vi "LowMaster.vi"() -> ()   [LabVIEW 2019]
uses:
  Ctl/tree.ctl
  Ctl/commands.ctl
  Ctl/Data Acquisition System.ctl
  Ctl/magnet.ctl
  Ctl/option.ctl
  <vilib>/Utility/file.llb/Write To Spreadsheet File (string).vi
panel:
  in  "Tab Control":T1(tab)
  in  "list":i32[](listbox)=[0]
  in  "Run":bool caption="Run/Stop"
  in  "open":bool
  in  "save":bool
  in  "copy 2":bool
  in  "paste":bool
  in  "delete":bool
  in  "clear":bool
  in  "Replace":bool
  in  "Update Sequence":bool
  in  "Tree":T2
  in  "line from":i32 caption="from line #" min=0
  out "log":i32[](listbox)
  in  "log save":bool
  in  "stop":bool
  out "Numeric":i32
  in  "Magnet":T3=enum."Cell8"
  in  "Data Acq":T4=enum."NML Data Acquisition-New.vi"
  in  "Quit LowMaster":bool
  out "current":i32
  in  "command":T5=enum."Comments"
  out "copy":string[][](array[string])
  # "Low Master 2016NT"
  # "Sequence Control Program   (contact: Ju-Hyun Park   JHPARK@magnet.fsu.edu)"
  # "Powered by MagLab"
  # "Magnet"
  # "QUIT LowMaster"
  # "Data Acquisition:"
  # "It doesn't hurt."
  # "Run/Stop"
  # "Sequence File"
  # "Sequence Edit Tool"
  # "* By default the log file is saved at the end of each run in the data folder."
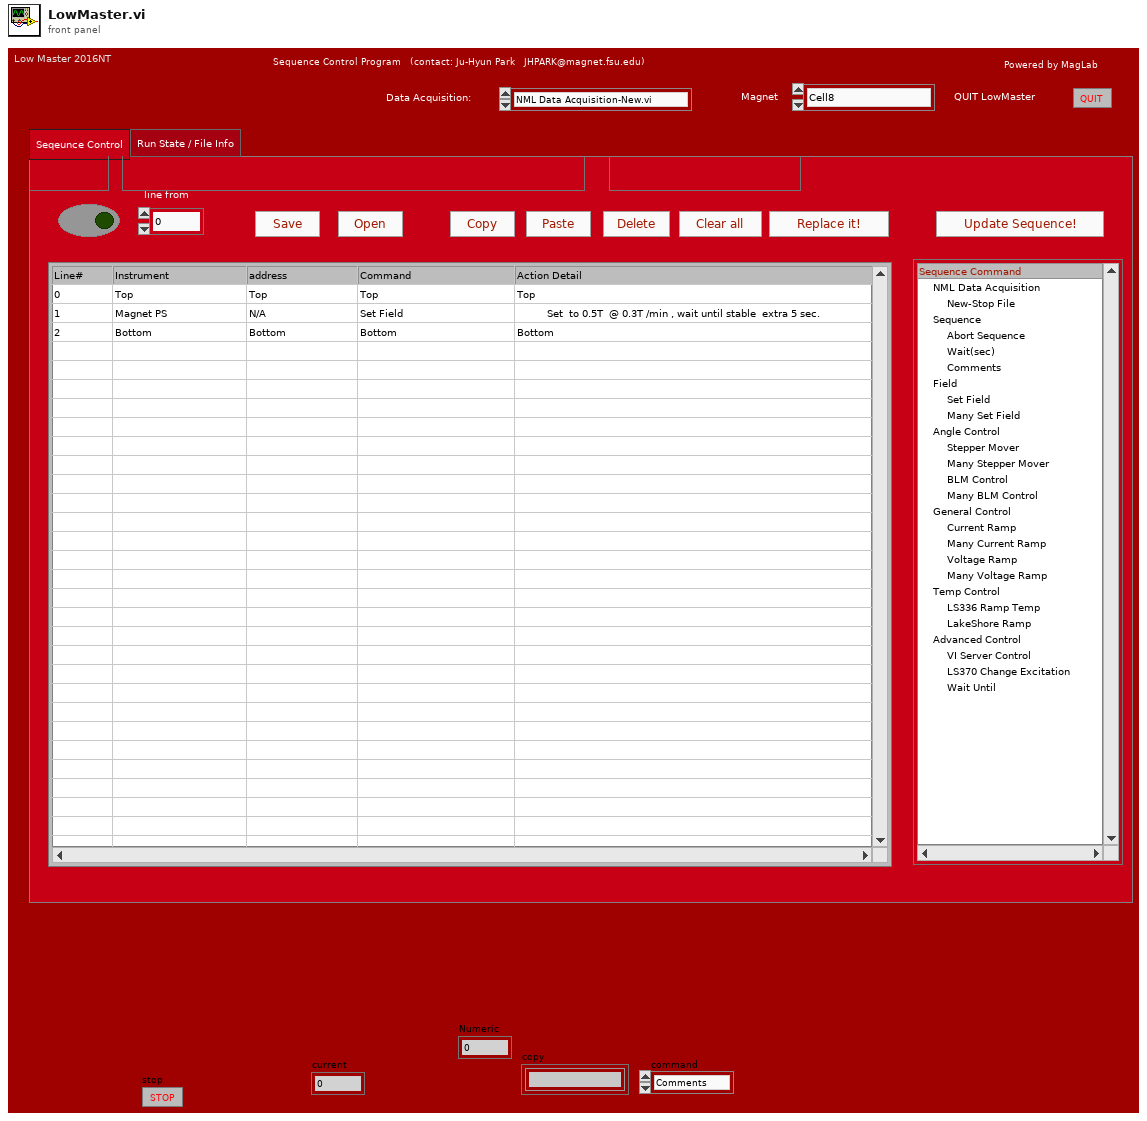
[diagram p1: front panel]
types:
  T1 = enum32{"Seqeunce Control", "Run State / File Info"}
  T2 = typedef "tree.ctl" = string[]
  T3 = typedef "magnet.ctl" = enum16{"SCM1", "SCM2", "SCM3", "SCMX", "Cell8", "Cell9", "Cell12", "Hybrid", "Great Magnet"}
  T4 = typedef "Data Acquisition System.ctl" = enum16{"NML Data Acquisition-old.vi", "NML Data Acquisition-New.vi"}
  T5 = typedef "commands.ctl" = enum16{"Voltage Ramp", "Many Voltage Ramp", "Current Ramp", "Many Current Ramp", "Comments", "Set Field", "Many Set Field", "Abort Sequence", "New-Stop File", "Wait(sec)", "BLM Control", "Many BLM Control", "Stepper Mover", "Many Stepper Mover", "LS336 Ramp Temp", "LakeShore Ramp", "VI Server Control", "LS370 Change Excitation", "Wait Until", "Nothing"}
  T6 = enum8{"Enabled", "Disabled", "Disabled and Grayed Out"}
  T7 = typedef "option.ctl" = enum16{"Tree", "List"}
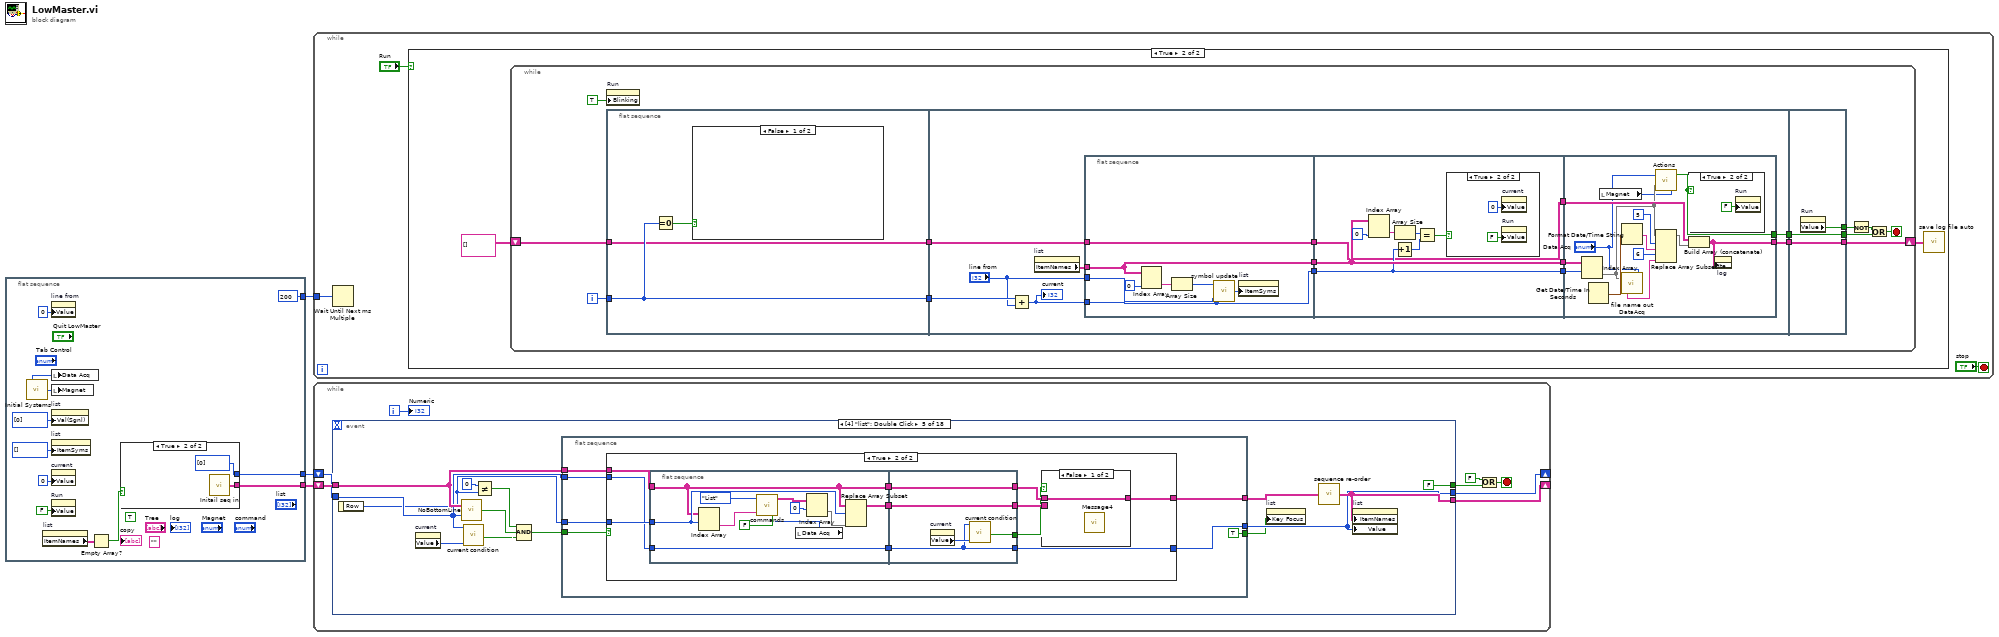
[diagram p0: block diagram]
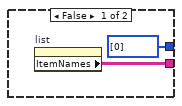
[diagram p2: hidden frame]
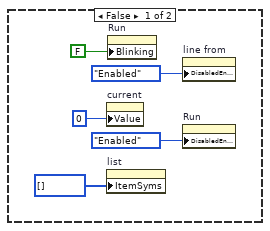
[diagram p3: hidden frame]
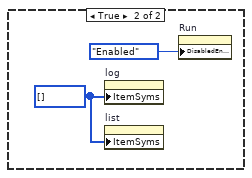
[diagram p4: hidden frame]
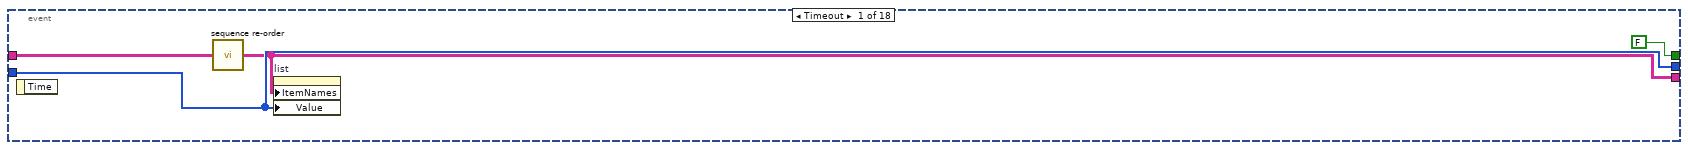
[diagram p7: hidden frame]
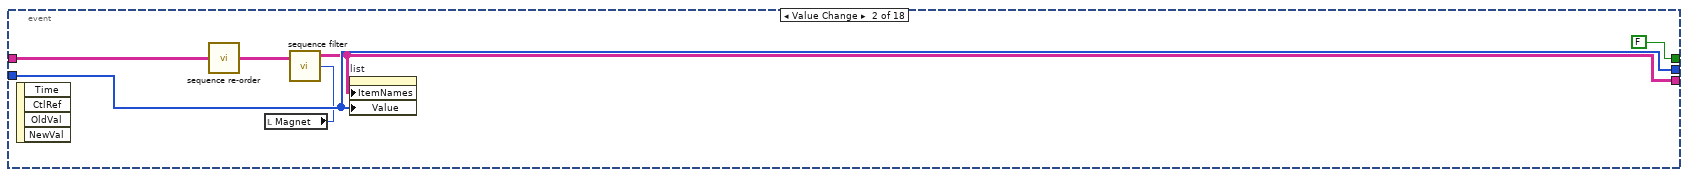
[diagram p8: hidden frame]
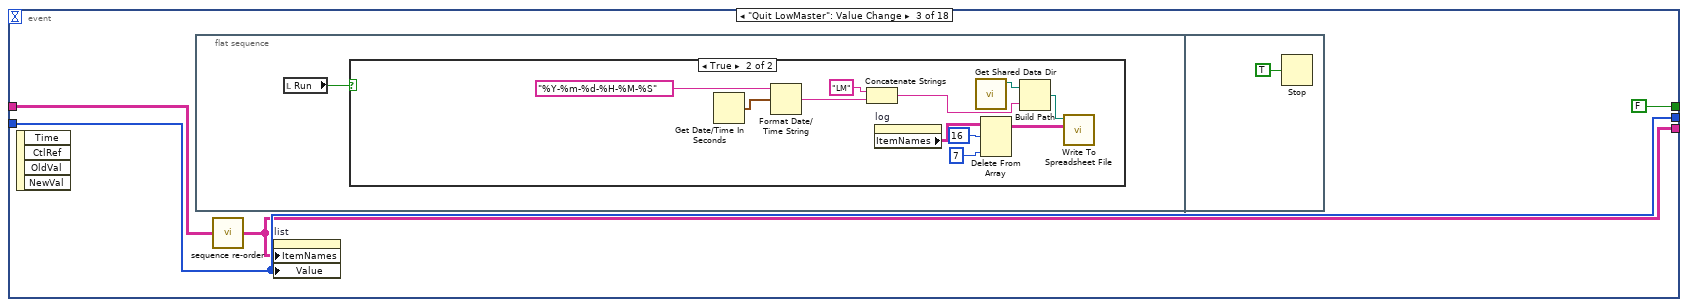
[diagram p9: hidden frame]
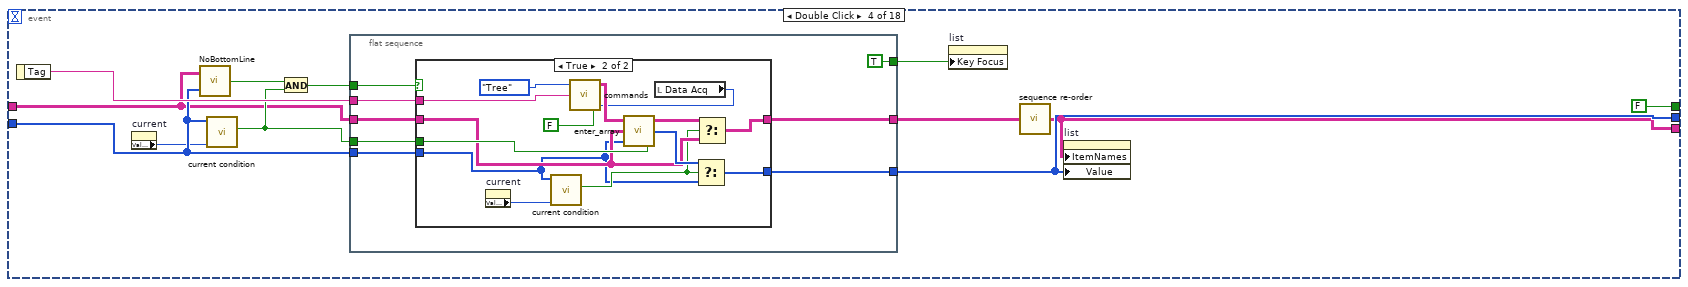
[diagram p11: hidden frame]
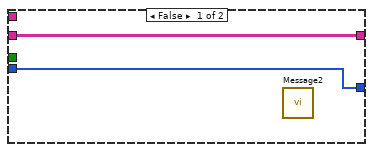
[diagram p12: hidden frame]
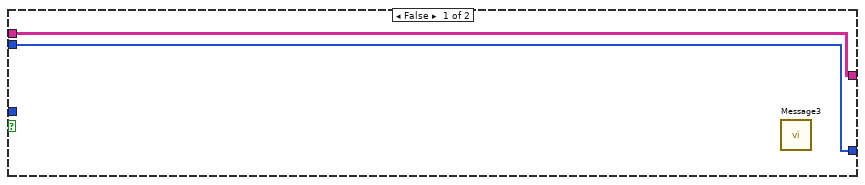
[diagram p13: hidden frame]
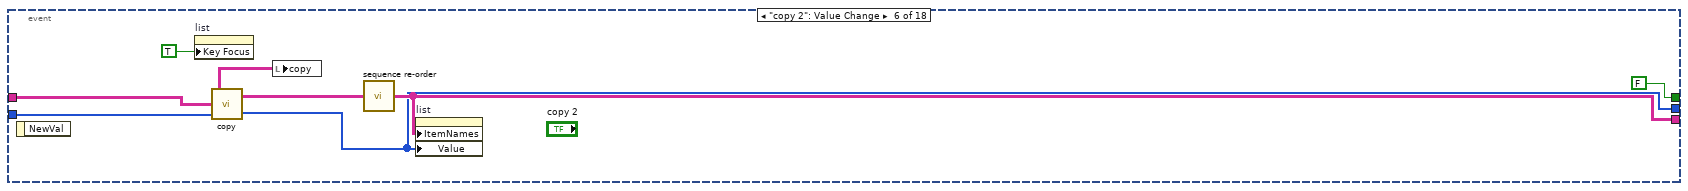
[diagram p15: hidden frame]
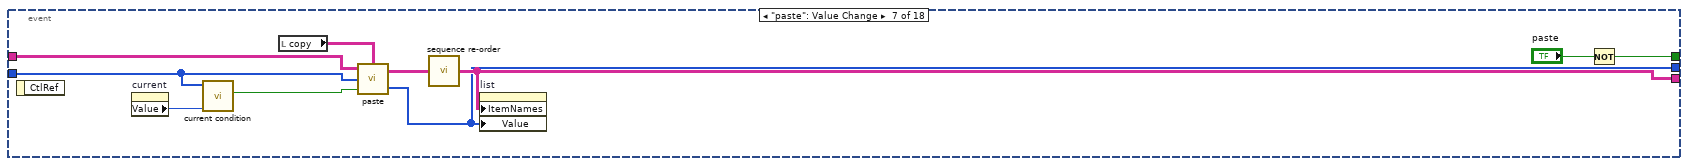
[diagram p16: hidden frame]
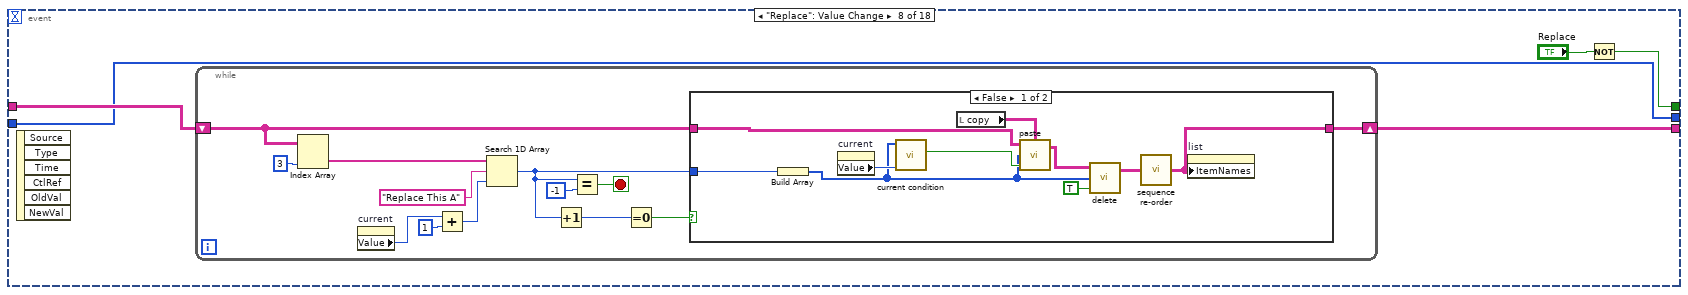
[diagram p17: hidden frame]
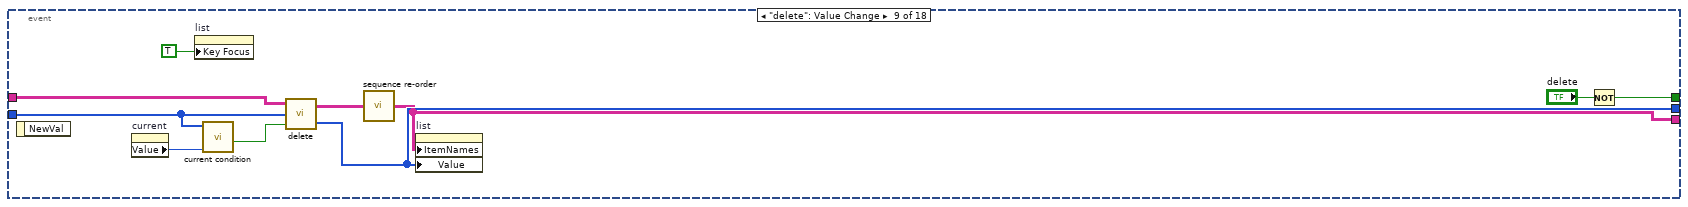
[diagram p19: hidden frame]
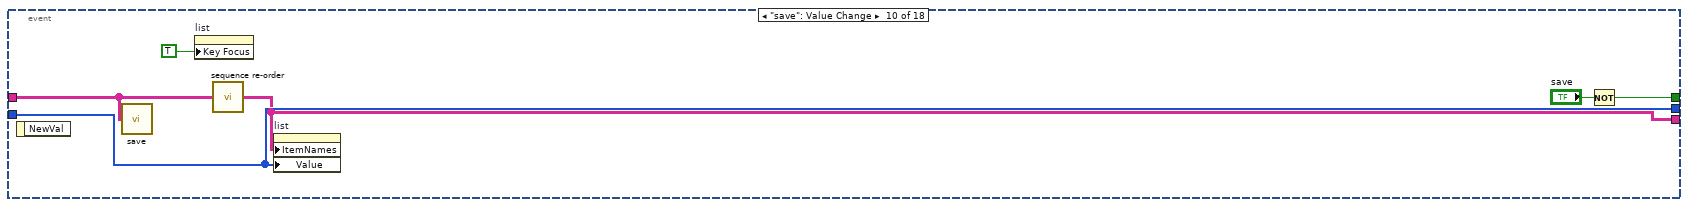
[diagram p20: hidden frame]
diagram:
  n1 = flat-sequence {
    tunnel: [w13] -> w3
    tunnel: [w12] -> w2
    tunnel: [u32 200 ("millisecond multiple")] -> w1
    frame #0 {
      (unwired) TRUE ("Monitor")
      (unwired) "" ("Start time str")
      n2 = call "Initial Systems.vi"() -> ("Magnet 2"=w4:T3, "Data Acq 2"=w5:T4)
      n3 = property on="list" class="MCListbox (strict)"() -> ("ItemNames"=w15:string[][])  [unwired: 2 in, 2 out]
      n4 = property on="line from" class="DigNum (strict)"("Value"=0 ("line")) -> ()  [unwired: 2 in, 2 out]
      n5 = local write "Data Acq"(w5) -> ()
      n6 = local write "Magnet"(w4) -> ()
      n7 = property on="list" class="MCListbox (strict)"("Val(Sgnl)"=i32[] [0] ("Value (Signaling)")) -> ()  [unwired: 2 in, 2 out]
      n8 = property on="list" class="MCListbox (strict)"("ItemSyms"=i32[] [] ("Item Symbols")) -> ()  [unwired: 2 in, 2 out]
      n9 = property on="current" class="DigNum (strict)"("Value"=0 ("current")) -> ()  [unwired: 2 in, 2 out]
      n10 = property on="Run" class="Bool (strict)"("Value"=FALSE ("Run")) -> ()  [unwired: 2 in, 2 out]
      n11 = Empty Array?(array=w15) -> (empty?=w14:bool)
      n12 = case shown="True" w14 {
        tunnel: [w17 w19] -> w13
        tunnel: [i32[] [0] ("Value (Signaling)") i32[] [0] ("Value (Signaling)")] -> w12
        frame False {
          n13 = property on="list" class="MCListbox (strict)"() -> ("ItemNames"=w17:string[][])  [unwired: 2 in, 2 out]
        }
        frame True {
          n14 = call "Initail seq in.vi"() -> ("INI seq in"=w19:string[][])
        }
      }
    }
  }
  n15 = while {
    tunnel: w1 -> [w20]
    stop <- "stop" stop-if-true
    n16 = Wait Until Next ms Multiple(millisecond multiple=w20) -> ()  [unwired: 1 out]
    n17 = case shown="True" "Run" {
      frame False {
        n18 = property on="current" class="DigNum (strict)"("Value"=0 ("current")) -> ()  [unwired: 2 in, 2 out]
        n19 = property on="list" class="MCListbox (strict)"("ItemSyms"=i32[] [] ("Item Symbols")) -> ()  [unwired: 2 in, 2 out]
        n20 = property on="Run" class="Bool (strict)"("Blinking"=FALSE) -> ()  [unwired: 2 in, 2 out]
        n21 = property on="line from" class="DigNum (strict)"("DisabledEnum"=T6."Enabled" ("Disabled")) -> ()  [unwired: 2 in, 2 out]
        n22 = property on="Run" class="Bool (strict)"("DisabledEnum"=T6."Enabled" ("Disabled")) -> ()  [unwired: 2 in, 2 out]
      }
      frame True {
        n23 = while {
          shift-right: [w35] -> w28
          shift-left: string[][] [] -> [w39]
          i -> [w41]
          stop <- w37 stop-if-true
          n24 = flat-sequence {
            tunnel: w41 -> [w44]
            tunnel: [w44] -> w33
            tunnel: w39 -> [w42]
            tunnel: [w42] -> w32
            tunnel: w33 -> [w59]
            tunnel: w32 -> [w56]
            tunnel: [w55] -> w31
            tunnel: [w54] -> w30
            tunnel: [w95] -> w40
            tunnel: [w94] -> w35
            tunnel: w31 -> [w94]
            tunnel: [w93] -> w36
            tunnel: w30 -> [w93]
            frame #0 {
              n25 = Equal To 0?(x=w44) -> (x = 0?=w43:bool)
              n26 = case shown="False" w43 {
                frame False {
                }
                frame True {
                  w45 = i32[] [] ("Item Symbols")
                  n27 = property on="log" class="MCListbox (strict)"("ItemSyms"=w45) -> ()  [unwired: 2 in, 2 out]
                  n28 = property on="list" class="MCListbox (strict)"("ItemSyms"=w45) -> ()  [unwired: 2 in, 2 out]
                  n29 = property on="Run" class="Bool (strict)"("DisabledEnum"=T6."Enabled" ("Disabled")) -> ()  [unwired: 2 in, 2 out]
                }
              }
            }
            frame #1 {
              n30 = Add(x=w59, y="line from") -> (x+y=w57:i32)
              "current" <- w57
              n31 = property on="list" class="MCListbox (strict)"() -> ("ItemNames"=w53:string[][])  [unwired: 2 in, 2 out]
              n32 = flat-sequence {
                tunnel: w57 -> [w64]
                tunnel: [w64] -> w52
                tunnel: w53 -> [w62]
                tunnel: [w62] -> w51
                tunnel: "line from" -> [w63]
                tunnel: w56 -> [w60]
                tunnel: [w60] -> w50
                tunnel: w52 -> [w70]
                tunnel: [w70] -> w49
                tunnel: w51 -> [w75]
                tunnel: [w75] -> w48
                tunnel: w50 -> [w68]
                tunnel: [w68] -> w47
                tunnel: w49 -> [w90]
                tunnel: w48 -> [w91]
                tunnel: w47 -> [w87]
                tunnel: [w85] -> w55
                tunnel: [w80] -> w54
                frame #0 {
                  n33 = Index Array(array=w62, index (col)=0 ("disabled index (col)")) -> (element=w66:string[])  [unwired: 1 in]
                  n34 = Array Size(array=w66) -> (size(s)=w65:i32)
                  n35 = call "symbol update.vi"("from index"=w63, "current"=w64, "total row"=w65) -> ("symbol"=w61:i32[])
                  n36 = property on="list" class="MCListbox (strict)"("ItemSyms"=w61) -> ()  [unwired: 2 in, 2 out]
                }
                frame #1 {
                  n37 = Index Array(array=w75, index (col)=0 ("disabled index (col)")) -> (element=w73:string[])  [unwired: 1 in]
                  n38 = Array Size(array=w73) -> (size(s)=w72:i32)
                  n39 = Increment(x=w70) -> (x+1=w69:i32)
                  n40 = Equal?(x=w72, y=w69) -> (x = y?=w71:bool)
                  n41 = case shown="True" w71 {
                    frame False {
                    }
                    frame True {
                      n42 = property on="current" class="DigNum (strict)"("Value"=0 ("current")) -> ()  [unwired: 2 in, 2 out]
                      n43 = property on="Run" class="Bool (strict)"("Value"=FALSE ("Run")) -> ()  [unwired: 2 in, 2 out]
                    }
                  }
                }
                frame #2 {
                  n44 = Index Array(array=w91, index (row)=w90) -> (element=w81:string[])  [unwired: 1 in]
                  n45 = Get Date/Time In Seconds() -> (seconds since 1Jan1904=w88:timestamp)
                  n46 = local read "Magnet"() -> (w78:T3)
                  n47 = Format Date/Time String(seconds (now)=w88) -> (date/time string=w83:string)  [unwired: 2 in]
                  n48 = call "file name out DataAcq.vi"("Data Acq"="Data Acq", "command text in"=w81) -> ("file name out"=w82:string)  [unwired: 1 in]
                  n49 = call "Actions.vi"("Magnet"=w78, "Array"=w81, "Data Acq"="Data Acq") -> ("Abort"=w80:bool)
                  n50 = Replace Array Subset(array=w81, new element #1=w83, index #1=5 ("index"), new element #2=w82, index #2=6 ("index")) -> (w86:string[])
                  n51 = case shown="True" w80 {
                    frame False {
                    }
                    frame True {
                      n52 = property on="Run" class="Bool (strict)"("Value"=FALSE ("Run")) -> ()  [unwired: 2 in, 2 out]
                    }
                  }
                  n53 = Build Array (concatenate)(w87, w86) -> (w85:string[][])
                  n54 = property on="log" class="MCListbox (strict)"("ItemNames"=w85) -> ()  [unwired: 2 in, 2 out]
                }
              }
            }
            frame #2 {
              n55 = property on="Run" class="Bool (strict)"() -> ("Value"=w95:bool)  [unwired: 2 in, 2 out]
            }
          }
          n56 = property on="Run" class="Bool (strict)"("Blinking"=TRUE) -> ()  [unwired: 2 in, 2 out]
          n57 = Not(x=w40) -> (.not. x?=w38:bool)
          n58 = Or(x=w38, y=w36) -> (x .or. y?=w37:bool)
        }
        n59 = call "save log file auto.vi"("log array"=w28) -> ()
      }
    }
  }
  n60 = while {
    shift-right: [w96] -> _
    shift-left: w3 -> [w101]
    shift-right: [w99] -> _
    shift-left: w2 -> [w100]
    i -> [w98]
    stop <- w102 stop-if-true
    n61 = event shown="[4] \"list\": Double Click" {
      selector: _ -> [_ _ _ _ _ _ _ _ _ _ _ _ _ _ _ _ _ _]
      dyn-events: _ -> [_ _ _ _ _ _ _ _ _ _ _ _ _ _ _ _ _ _]
      timeout: _ -> [_ _ _ _ _ _ _ _ _ _ _ _ _ _ _ _ _ _]
      tunnel: w101 -> [w105 w111 w115 w135 w178 w226 w234 w239 w275 w277 w283 w296 w307 w344 w348 w373 w376 _]
      tunnel: [w104 w110 w114 w132 w169 w220 w228 w238 w266 w276 w282 w291 w298 w343 w349 w369 w375 w387] -> w96
      tunnel: [FALSE FALSE FALSE FALSE FALSE FALSE w235 w240 w273 w280 w290 w295 FALSE FALSE FALSE w367 FALSE w391] -> w103
      tunnel: w100 -> [w106 w112 w116 w137 w175 w225 w232 w237 w270 w278 w284 w293 w303 _ w350 w370 w377 _]
      tunnel: [w106 w112 w116 w134 w168 w219 w227 w237 w268 w278 w284 w293 w300 w345 w350 w370 w377 w389] -> w99
      event Timeout {
        n62 = event-data() -> ()  [unwired: 1 in, 1 out]
        n63 = call "sequence re-order.vi"("seq in"=w105) -> ("seq out"=w104:string[][])
        n64 = property on="list" class="MCListbox (strict)"("ItemNames"=w104, "Value"=w106) -> ()  [unwired: 2 in, 2 out]
      }
      event Value Change {
        n65 = event-data() -> ()  [unwired: 1 in, 4 out]
        n66 = call "sequence re-order.vi"("seq in"=w111) -> ("seq out"=w109:string[][])
        n67 = local read "Magnet"() -> (w108:T3)
        n68 = call "sequence filter.vi"("seq in"=w109, "Magnet"=w108) -> ("seq  out"=w110:string[][])  [unwired: 2 in]
        n69 = property on="list" class="MCListbox (strict)"("ItemNames"=w110, "Value"=w112) -> ()  [unwired: 2 in, 2 out]
      }
      event "Quit LowMaster": Value Change {
        n70 = event-data() -> ()  [unwired: 1 in, 4 out]
        n71 = flat-sequence {
          frame #0 {
            n72 = local read "Run"() -> (w118:bool)
            n73 = case shown="True" w118 {
              frame False {
              }
              frame True {
                n74 = Get Date/Time In Seconds() -> (seconds since 1Jan1904=w127:timestamp)
                n75 = Format Date/Time String(time format string (%c)="%Y-%m-%d-%H-%M-%S", seconds (now)=w127) -> (date/time string=w129:string)  [unwired: 1 in]
                n76 = Concatenate Strings("LM" ("string"), w129) -> (w125:string)
                n77 = property on="log" class="MCListbox (strict)"() -> ("ItemNames"=w119:string[][])  [unwired: 2 in, 2 out]
                n78 = call "Get Shared Data Dir.vi"() -> ("Data Directory Path"=w124:path)  [unwired: 2 in, 1 out]
                n79 = Delete From Array(array=w119, length=16 ("disabled index (col)"), index (col)=7 ("disabled index (col)")) -> (array with subset deleted=w121:string[][])  [unwired: 1 in, 1 out]
                n80 = Build Path(base path=w124, name or relative path=w125) -> (appended path=w126:path)
                n81 = call-poly <vilib>:"Write To Spreadsheet File.vi"("2D data"=w121, "file path (dialog if empty)"=w126) -> ()  [unwired: 6 in, 1 out]
              }
            }
          }
          frame #1 {
            n82 = Stop(stop? (T)=TRUE) -> ()
          }
        }
        n83 = call "sequence re-order.vi"("seq in"=w115) -> ("seq out"=w114:string[][])
        n84 = property on="list" class="MCListbox (strict)"("ItemNames"=w114, "Value"=w116) -> ()  [unwired: 2 in, 2 out]
      }
      event Double Click {
        n85 = event-data() -> ("Tag"=w141:string)  [unwired: 1 in]
        n86 = property on="current" class="DigNum (strict)"() -> ("Value"=w136:i32)  [unwired: 2 in, 2 out]
        n87 = call "NoBottomLine.vi"("Value in"=w137, "ItemNames in"=w135) -> ("no bottom?"=w139:bool)
        n88 = call "current condition.vi"("current"=w136, "list value"=w137) -> ("oneminus"=w138:bool)  [unwired: 1 out]
        n89 = And(x=w139, y=w138) -> (x .and. y?=w142:bool)
        n90 = flat-sequence {
          tunnel: w142 -> [w149]
          tunnel: w141 -> [w148]
          tunnel: w135 -> [w146]
          tunnel: w137 -> [w145]
          tunnel: w138 -> [w144]
          tunnel: [w150] -> w133
          tunnel: [w147] -> w134
          tunnel: [TRUE ("Key Focus")] -> w131
          frame #0 {
            n91 = case shown="True" w149 {
              tunnel: [w152 w161] -> w150
              tunnel: w145 -> [w151 w159]
              tunnel: [w151 w158] -> w147
              tunnel: w144 -> [_ w166]
              tunnel: w146 -> [w152 w162]
              tunnel: w148 -> [_ w165]
              frame False {
                n92 = call "Message2"() -> ()  [unwired: 10 in, 2 out]
              }
              frame True {
                n93 = property on="current" class="DigNum (strict)"() -> ("Value"=w154:i32)  [unwired: 2 in, 2 out]
                n94 = call "current condition.vi"("current"=w154, "list value"=w159) -> ("oneminus"=w160:bool)  [unwired: 1 out]
                n95 = local read "Data Acq"() -> (w153:T4)
                n96 = call "commands.vi"("Data Acq"=w153, "Scan Seq?"=FALSE, "tree com"=w165, "option"=option."Tree") -> ("output"=w157:string[][])  [unwired: 1 in]
                n97 = call "enter_array.vi"("future?"=w166, "Cursor IN"=w159, "ItemNames in"=w162, "array"=w157) -> ("Cursor OUT"=w164:i32[], "ItemNames out"=w163:string[][])
                n98 = Select(t=w164, s=w160, f=w159) -> (s? t:f=w158:i32[])
                n99 = Select(t=w163, s=w160, f=w162) -> (s? t:f=w161:string[][])
              }
            }
          }
        }
        n100 = property on="list" class="MCListbox (strict)"("Key Focus"=w131) -> ()  [unwired: 2 in, 2 out]
        n101 = call "sequence re-order.vi"("seq in"=w133) -> ("seq out"=w132:string[][])
        n102 = property on="list" class="MCListbox (strict)"("ItemNames"=w132, "Value"=w134) -> ()  [unwired: 2 in, 2 out]
      }
      event "list": Double Click {
        n103 = event-data() -> ("Row"=w172:i32)  [unwired: 1 in]
        n104 = property on="current" class="DigNum (strict)"() -> ("Value"=w176:i32)  [unwired: 2 in, 2 out]
        n105 = call "NoBottomLine.vi"("Value in"=w175, "ItemNames in"=w178) -> ("no bottom?"=w177:bool)
        n106 = call "current condition.vi"("current"=w176, "list value"=w175) -> ("direct"=w174:bool)  [unwired: 1 out]
        n107 = Not Equal?(x=0 ("y"), y=w172) -> (x != y?=w180:bool)
        n108 = Compound Arithmetic op=AND(w180, w177, w174) -> (w179:bool)
        n109 = flat-sequence {
          tunnel: w178 -> [w187]
          tunnel: w172 -> [w185]
          tunnel: w179 -> [w183]
          tunnel: w175 -> [w182]
          tunnel: [w186] -> w170
          tunnel: [w184] -> w168
          tunnel: [TRUE ("Key Focus")] -> w167
          frame #0 {
            n110 = case shown="True" w183 {
              tunnel: w187 -> [w189 w200]
              tunnel: [w189 w198] -> w186
              tunnel: w185 -> [_ w199]
              tunnel: w182 -> [w188 w195]
              tunnel: [w188 w193] -> w184
              frame False {
                n111 = call "Message3"() -> ()  [unwired: 10 in, 2 out]
              }
              frame True {
                n112 = flat-sequence {
                  tunnel: w200 -> [w207]
                  tunnel: [w209] -> w192
                  tunnel: w199 -> [w208]
                  tunnel: [w207] -> w191
                  tunnel: w195 -> [w202]
                  tunnel: [w202] -> w190
                  tunnel: [w213] -> w197
                  tunnel: w192 -> [w213]
                  tunnel: [w212] -> w196
                  tunnel: w191 -> [w212]
                  tunnel: w190 -> [w214]
                  tunnel: [w215] -> w194
                  tunnel: [w214] -> w193
                  frame #0 {
                    n113 = Index Array(array=w207, index (row)=w208) -> (element=w203:string[])  [unwired: 1 in]
                    n114 = local read "Data Acq"() -> (w201:T4)
                    n115 = call "commands.vi"("Data Acq"=w201, "Scan Seq?"=FALSE, "list com"=w203, "option"=option."List") -> ("output"=w205:string[][])  [unwired: 1 in]
                    n116 = Index Array(array=w205, index (row)=0) -> (element=w210:string[])  [unwired: 1 in]
                    n117 = Replace Array Subset(array=w207, new element=w210, index (row)=w208) -> (w209:string[][])  [unwired: 1 in]
                  }
                  frame #1 {
                    n118 = property on="current" class="DigNum (strict)"() -> ("Value"=w216:i32)  [unwired: 2 in, 2 out]
                    n119 = call "current condition.vi"("current"=w216, "list value"=w214) -> ("direct"=w215:bool)  [unwired: 1 out]
                  }
                }
                n120 = case shown="False" w194 {
                  tunnel: [w217 w218] -> w198
                  tunnel: w197 -> [_ w218]
                  tunnel: w196 -> [w217 _]
                  frame False {
                    n121 = call "Message4"() -> ()  [unwired: 10 in, 2 out]
                  }
                  frame True {
                  }
                }
              }
            }
          }
        }
        n122 = property on="list" class="MCListbox (strict)"("Key Focus"=w167) -> ()  [unwired: 2 in, 2 out]
        n123 = call "sequence re-order.vi"("seq in"=w170) -> ("seq out"=w169:string[][])
        n124 = property on="list" class="MCListbox (strict)"("ItemNames"=w169, "Value"=w168) -> ()  [unwired: 2 in, 2 out]
      }
      event "copy 2": Value Change {
        n125 = event-data() -> ()  [unwired: 1 in, 1 out]
        n126 = property on="list" class="MCListbox (strict)"("Key Focus"=TRUE) -> ()  [unwired: 2 in, 2 out]
        n127 = call "copy.vi"("Value"=w225, "ItemNames in"=w226) -> ("val(sgnl)"=w219:i32[], "ItemNames out"=w221:string[][], "copyAry"=w224:string[][])
        n128 = local write "copy"(w224) -> ()
        n129 = call "sequence re-order.vi"("seq in"=w221) -> ("seq out"=w220:string[][])
        n130 = property on="list" class="MCListbox (strict)"("ItemNames"=w220, "Value"=w219) -> ()  [unwired: 2 in, 2 out]
      }
      event "paste": Value Change {
        n131 = event-data() -> ()  [unwired: 1 in, 1 out]
        n132 = property on="current" class="DigNum (strict)"() -> ("Value"=w230:i32)  [unwired: 2 in, 2 out]
        n133 = call "current condition.vi"("current"=w230, "list value"=w232) -> ("oneminus"=w231:bool)  [unwired: 1 out]
        n134 = local read "copy"() -> (w233:string[][])
        n135 = call "paste.vi"("copyAry"=w233, "future event?"=w231, "Value"=w232, "ItemNames in"=w234) -> ("val(sgnl)"=w227:i32[], "ItemNames out"=w229:string[][])
        n136 = call "sequence re-order.vi"("seq in"=w229) -> ("seq out"=w228:string[][])
        n137 = property on="list" class="MCListbox (strict)"("ItemNames"=w228, "Value"=w227) -> ()  [unwired: 2 in, 2 out]
        n138 = Not(x="paste") -> (.not. x?=w235:bool)
      }
      event "Replace": Value Change {
        n139 = event-data() -> ()  [unwired: 1 in, 6 out]
        n140 = while {
          shift-right: [w247] -> w238
          shift-left: w239 -> [w246]
          stop <- w248 stop-if-true
          n141 = Index Array(array=w246, index (col)=3 ("disabled index (col)")) -> (element=w245:string[])  [unwired: 1 in]
          n142 = property on="current" class="DigNum (strict)"() -> ("Value"=w252:i32)  [unwired: 2 in, 2 out]
          n143 = Add(x=w252, y=1) -> (x+y=w250:i32)
          n144 = Search 1D Array(1D array=w245, element="Replace This A", start index (0)=w250) -> (index of element=w243:i32)
          n145 = Increment(x=w243) -> (x+1=w244:i32)
          n146 = Equal?(x=w243, y=-1) -> (x = y?=w248:bool)
          n147 = Equal To 0?(x=w244) -> (x = 0?=w242:bool)
          n148 = case shown="False" w242 {
            tunnel: [w261 w265] -> w247
            tunnel: w246 -> [w260 w265]
            tunnel: w243 -> [w255 _]
            frame False {
              n149 = Build Array(w255) -> (w256:i32[])
              n150 = property on="current" class="DigNum (strict)"() -> ("Value"=w264:i32)  [unwired: 2 in, 2 out]
              n151 = call "current condition.vi"("current"=w264, "list value"=w256) -> ("oneminus"=w263:bool)  [unwired: 1 out]
              n152 = local read "copy"() -> (w262:string[][])
              n153 = call "paste.vi"("copyAry"=w262, "future event?"=w263, "Value"=w256, "ItemNames in"=w260) -> ("ItemNames out"=w259:string[][])  [unwired: 1 out]
              n154 = call "delete.vi"("future event?"=TRUE, "Value"=w256, "ItemNames in"=w259) -> ("ItemNames out"=w258:string[][])  [unwired: 1 out]
              n155 = call "sequence re-order.vi"("seq in"=w258) -> ("seq out"=w261:string[][])
              n156 = property on="list" class="MCListbox (strict)"("ItemNames"=w261) -> ()  [unwired: 2 in, 2 out]
            }
            frame True {
            }
          }
        }
        n157 = Not(x="Replace") -> (.not. x?=w240:bool)
      }
      event "delete": Value Change {
        n158 = event-data() -> ()  [unwired: 1 in, 1 out]
        n159 = property on="current" class="DigNum (strict)"() -> ("Value"=w269:i32)  [unwired: 2 in, 2 out]
        n160 = property on="list" class="MCListbox (strict)"("Key Focus"=TRUE) -> ()  [unwired: 2 in, 2 out]
        n161 = call "current condition.vi"("current"=w269, "list value"=w270) -> ("direct"=w271:bool)  [unwired: 1 out]
        n162 = call "delete.vi"("future event?"=w271, "Value"=w270, "ItemNames in"=w275) -> ("val(sgnl)"=w268:i32[], "ItemNames out"=w267:string[][])
        n163 = call "sequence re-order.vi"("seq in"=w267) -> ("seq out"=w266:string[][])
        n164 = property on="list" class="MCListbox (strict)"("ItemNames"=w266, "Value"=w268) -> ()  [unwired: 2 in, 2 out]
        n165 = Not(x="delete") -> (.not. x?=w273:bool)
      }
      event "save": Value Change {
        n166 = event-data() -> ()  [unwired: 1 in, 1 out]
        n167 = call "save.vi"("ItemNames"=w277) -> ()
        n168 = property on="list" class="MCListbox (strict)"("Key Focus"=TRUE) -> ()  [unwired: 2 in, 2 out]
        n169 = call "sequence re-order.vi"("seq in"=w277) -> ("seq out"=w276:string[][])
        n170 = property on="list" class="MCListbox (strict)"("ItemNames"=w276, "Value"=w278) -> ()  [unwired: 2 in, 2 out]
        n171 = Not(x="save") -> (.not. x?=w280:bool)
      }
      event "log save": Value Change {
        n172 = event-data() -> ()  [unwired: 1 in, 1 out]
        n173 = property on="log" class="MCListbox (strict)"() -> ("ItemNames"=w288:string[][])  [unwired: 2 in, 2 out]
        n174 = call "sequence re-order.vi"("seq in"=w283) -> ("seq out"=w282:string[][])
        n175 = property on="list" class="MCListbox (strict)"("ItemNames"=w282, "Value"=w284) -> ()  [unwired: 2 in, 2 out]
        n176 = Delete From Array(array=w288, length=16 ("disabled index (col)"), index (col)=7 ("disabled index (col)")) -> (array with subset deleted=w285:string[][])  [unwired: 1 in, 1 out]
        n177 = call "save.vi"("ItemNames"=w285) -> ()
        n178 = Not(x="log save") -> (.not. x?=w290:bool)
      }
      event "open": Value Change {
        n179 = event-data() -> ()  [unwired: 1 in, 1 out]
        n180 = property on="list" class="MCListbox (strict)"("Key Focus"=TRUE) -> ()  [unwired: 2 in, 2 out]
        n181 = call "open.vi"("ItemNames in"=w296) -> ("ItemNames out"=w292:string[][])
        n182 = call "sequence re-order.vi"("seq in"=w292) -> ("seq out"=w291:string[][])
        n183 = property on="list" class="MCListbox (strict)"("ItemNames"=w291, "Value"=w293) -> ()  [unwired: 2 in, 2 out]
        n184 = Not(x="open") -> (.not. x?=w295:bool)
      }
      event "list": Key Down {
        n185 = event-data() -> ("PlatMods.Cmd"=w310:bool, "PlatMods.Ctrl"=w309:bool, "ScanCode"=w301:i16)  [unwired: 1 in]
        n186 = property on="current" class="DigNum (strict)"() -> ("Value"=w302:i32)  [unwired: 2 in, 2 out]
        n187 = Or(x=w310, y=w309) -> (x .or. y?=w308:bool)
        n188 = call "current condition.vi"("current"=w302, "list value"=w303) -> ("direct"=w304:bool, "oneminus"=w305:bool)
        n189 = case shown="False" w308 {
          tunnel: w301 -> [w316 w329]
          tunnel: w307 -> [w315 w328]
          tunnel: [w314 w327] -> w299
          tunnel: w303 -> [w312 w326]
          tunnel: w305 -> [_ w325]
          tunnel: w304 -> [w313 _]
          tunnel: [w311 w324] -> w300
          frame False {
            n190 = case shown="0, Default" w316 {
              tunnel: w315 -> [w318 w323]
              tunnel: [w318 w322] -> w314
              tunnel: w313 -> [_ w321]
              tunnel: w312 -> [_ w320]
              tunnel: [w317 w319] -> w311
              frame 0, Default {
                n191 = property on="list" class="MCListbox (strict)"() -> ("Value"=w317:i32[])  [unwired: 2 in, 2 out]
              }
              frame 51 {
                n192 = call "delete.vi"("future event?"=w321, "Value"=w320, "ItemNames in"=w323) -> ("val(sgnl)"=w319:i32[], "ItemNames out"=w322:string[][])
              }
            }
          }
          frame True {
            n193 = case shown="0, Default" w329 {
              tunnel: w328 -> [w331 w336 w342]
              tunnel: [w331 w335 w339] -> w327
              tunnel: w326 -> [_ w333 w341]
              tunnel: w325 -> [_ _ w338]
              tunnel: [w330 w332 w337] -> w324
              frame 0, Default {
                n194 = property on="list" class="MCListbox (strict)"() -> ("Value"=w330:i32[])  [unwired: 2 in, 2 out]
              }
              frame 8 {
                n195 = call "copy.vi"("Value"=w333, "ItemNames in"=w336) -> ("val(sgnl)"=w332:i32[], "ItemNames out"=w335:string[][], "copyAry"=w334:string[][])
                n196 = local write "copy"(w334) -> ()
              }
              frame 9 {
                n197 = local read "copy"() -> (w340:string[][])
                n198 = call "paste.vi"("copyAry"=w340, "future event?"=w338, "Value"=w341, "ItemNames in"=w342) -> ("val(sgnl)"=w337:i32[], "ItemNames out"=w339:string[][])
              }
            }
          }
        }
        n199 = call "sequence re-order.vi"("seq in"=w299) -> ("seq out"=w298:string[][])
        n200 = property on="list" class="MCListbox (strict)"("ItemNames"=w298, "Value"=w300) -> ()  [unwired: 2 in, 2 out]
      }
      event "list": Value Change {
        n201 = event-data() -> ("NewVal"=w345:i32[])  [unwired: 1 in]
        n202 = call "sequence re-order.vi"("seq in"=w344) -> ("seq out"=w343:string[][])
        n203 = property on="list" class="MCListbox (strict)"("ItemNames"=w343, "Value"=w345) -> ()  [unwired: 2 in, 2 out]
      }
      event "Run": Value Change {
        n204 = event-data() -> ("NewVal"=w358:bool)  [unwired: 1 in]
        n205 = call "sequence re-order.vi"("seq in"=w348) -> ()  [unwired: 1 out]
        n206 = local read "Magnet"() -> (w347:T3)
        n207 = property on="line from" class="DigNum (strict)"() -> ("Value"=w352:i32)  [unwired: 2 in, 2 out]
        n208 = Array Size(array=w348) -> (size(s)=w353:i32[])
        n209 = call "sequence filter.vi"("seq in"=w348, "Magnet"=w347) -> ("seq  out"=w349:string[][])  [unwired: 2 in]
        n210 = property on="list" class="MCListbox (strict)"("ItemNames"=w349, "Value"=w350) -> ()  [unwired: 2 in, 2 out]
        n211 = Increment(x=w352) -> (x+1=w356:i32)
        n212 = Index Array(array=w353, index=0) -> (element=w355:i32)
        n213 = Greater Or Equal?(x=w356, y=w355) -> (x >= y?=w351:bool)
        n214 = case shown="True" w358 {
          tunnel: w351 -> [_ w362]
          frame False {
            n215 = property on="list" class="MCListbox (strict)"("Val(Sgnl)"=i32[] [0] ("Value (Signaling)")) -> ()  [unwired: 2 in, 2 out]
            n216 = property on="Run" class="Bool (strict)"("DisabledEnum"=T6."Disabled and Grayed Out" ("Disabled")) -> ()  [unwired: 2 in, 2 out]
            n217 = One Button Dialog(message="will stop after current line") -> ()  [unwired: 1 in, 1 out]
          }
          frame True {
            n218 = case shown="False" w362 {
              frame False {
                n219 = property on="list" class="MCListbox (strict)"("Val(Sgnl)"=i32[] [0] ("Value (Signaling)")) -> ()  [unwired: 2 in, 2 out]
                n220 = property on="line from" class="DigNum (strict)"("DisabledEnum"=T6."Disabled and Grayed Out" ("Disabled")) -> ()  [unwired: 2 in, 2 out]
              }
              frame True {
                n221 = property on="Run" class="Bool (strict)"("Value"=FALSE ("Run")) -> ()  [unwired: 2 in, 2 out]
                n222 = One Button Dialog(message="The line # is greater than \nsequence itself.") -> ()  [unwired: 1 in, 1 out]
              }
            }
          }
        }
      }
      event "Update Sequence": Value Change {
        n223 = event-data() -> ()  [unwired: 1 in, 6 out]
        n224 = call "sequence re-order.vi"("seq in"=w373) -> ("seq out"=w372:string[][])
        n225 = local read "Magnet"() -> (w371:T3)
        n226 = call "sequence filter.vi"("seq in"=w372, "Magnet"=w371) -> ("seq  out"=w369:string[][])  [unwired: 2 in]
        n227 = property on="list" class="MCListbox (strict)"("ItemNames"=w369) -> ()  [unwired: 2 in, 2 out]
        n228 = Not(x="Update Sequence") -> (.not. x?=w367:bool)
      }
      event "line from": Value Change {
        n229 = event-data() -> ("NewVal"=w378:i32)  [unwired: 1 in]
        n230 = property on="list" class="MCListbox (strict)"("Val(Sgnl)"=w377) -> ()  [unwired: 2 in, 2 out]
        n231 = property on="list" class="MCListbox (strict)"("Key Focus"=TRUE) -> ()  [unwired: 2 in, 2 out]
        n232 = Array Size(array=w376) -> (size(s)=w384:i32[])
        n233 = call "sequence re-order.vi"("seq in"=w376) -> ("seq out"=w375:string[][])
        n234 = property on="list" class="MCListbox (strict)"("ItemNames"=w375, "Value"=w377) -> ()  [unwired: 2 in, 2 out]
        n235 = Increment(x=w378) -> (x+1=w382:i32)
        n236 = Index Array(array=w384, index=0) -> (element=w381:i32)
        n237 = Greater Or Equal?(x=w382, y=w381) -> (x >= y?=w380:bool)
        n238 = case shown="True" w380 {
          frame False {
          }
          frame True {
            n239 = property on="line from" class="DigNum (strict)"("Val(Sgnl)"=0) -> ()  [unwired: 2 in, 2 out]
            n240 = One Button Dialog(message="The line # is greater than \nsequence itself.") -> ()  [unwired: 1 in, 1 out]
          }
        }
      }
      event "clear": Value Change {
        w389 = i32[] [0] ("Value (Signaling)")
        n241 = event-data() -> ()  [unwired: 1 in, 4 out]
        n242 = call "Initail seq in.vi"() -> ("INI seq in"=w388:string[][])
        n243 = call "sequence re-order.vi"("seq in"=w388) -> ("seq out"=w387:string[][])
        n244 = property on="list" class="MCListbox (strict)"("ItemNames"=w387, "Value"=w389) -> ()  [unwired: 2 in, 2 out]
        n245 = Not(x="clear") -> (.not. x?=w391:bool)
      }
    }
    n246 = Or(x=FALSE, y=w103) -> (x .or. y?=w102:bool)
    "Numeric" <- w98
  }
